vi "Measure IV AC.vi"(0 "IV Sampling":enum16{"Linear", "Logartihmic"}(ring)=enum."Logartihmic", 1 "6221 Address":string="12", 2 "SR860 Address":string="4", 5 "IV Type":T5(ring), 7 "dI or Imin":dbl=1e-08, 9 "Imax":dbl=0.001, 11 "Ipts":i16=16, 12 "Frequency":string="1711", 13 "Filter BW":T4(ring)=enum."10 ms", 14 "Ch1 Harmonic":T3(ring)) -> (8 "Data array":dbl[][](array[numeric])=[[1e-08, 3.5543477267321877e-09, 1.0096080012560406e-09, 0.35543477267321877, 0.10096080012560406], [2.1544e-08, 8.03021465434206e-08, 1.4967572525627115e-09, 3.727355483820117, 0.06947443615682841], [4.6416e-08, 1.2554884259996513e-07, 1.0072382615044234e-09, 2.704861310754161, 0.021700238312315226], [1e-07, 2.84475994760669e-07, 3.281983319934282e-09, 2.84475994760669, 0.03281983319934282], [2.15443e-07, 5.927384150172799e-07, 1.8001529832205674e-09, 2.7512539976572916, 0.00835558817515801], [4.64159e-07, 1.3026465262022668e-06, 1.3744287256216488e-09, 2.8064661596613805, 0.002961116181355201], [1e-06, 2.7703576330750934e-06, 1.1115718058886643e-09, 2.7703576330750934, 0.0011115718058886644], [2.154e-06, 5.988217456120992e-06, 6.723626581805896e-10, 2.780045244253014, 0.00031214608086378346], [4.642e-06, 1.3094926590184741e-05, 5.81885584849347e-10, 2.820966520935963, 0.00012535234486198772], [1e-05, 2.7790200547883614e-05, 2.9330275661149422e-09, 2.779020054788361, 0.0002933027566114942], [2.1544e-05, 5.994770525319382e-05, 3.4220733482770047e-10, 2.7825707971218816, 1.5884113202176964e-05], [4.6416e-05, 0.00012909908491565147, 1.8729144160359265e-09, 2.7813487787756697, 4.035062082118077e-05], [0.0001, 0.0002775546062139256, 2.9235413634973257e-09, 2.775546062139256, 2.9235413634973255e-05], [0.000215443, 0.0005982162022064585, 3.75564815539695e-09, 2.776679688857185, 1.7432212489600265e-05], [0.000464159, 0.001288317614580592, 1.080391628779838e-09, 2.7755954631507564, 2.3276326189513462e-06], [0.001, 0.00277545716289751, 3.798989931589336e-09, 2.77545716289751, 3.798989931589336e-06]], 10 "Error 6221":errorcluster, 15 "Error SR860":errorcluster)   [LabVIEW 2020]
uses:
  <vilib>/Analysis/1siggen.llb/Ramp Pattern by Delta.vi
  <vilib>/Analysis/NI_AALBase.lvlib
panel:
  out "I-V Plot":cluster{"Ramp Pattern":dbl[], dbl[]}[](graph)
  in  "TRIG Wave":bool=TRUE
  out "V STD Now":dbl=3.798989931589336e-09
  out "V Mean Now":dbl=0.00277545716289751
  out "Garbage":errorcluster={"status"=TRUE, "code"=6, "source"="GPIB Read in Measure IV.vi"}
  out "Lockin Garbage":string
  in  "Buffer Size (kb)":i32=2
  out "Buffer":sgl[](array[numeric])=[0.0027754628, 9.413887, 0.0027754628, 9.413885, 0.0027754628, 9.413885, 0.0027754628, 9.413884, 0.0027754628, 9.413881, 0.0027754628, 9.413881, 0.0027754628, 9.41388, 0.0027754628, 9.413878, 0.0027754628, 9.413878, 0.0027754626, 9.4138775, 0.0027754626, 9.4138775, 0.0027754626, 9.413875, 0.0027754626, 9.413875, 0.0027754626, 9.413874, 0.0027754626, 9.413872, 0.0027754626, 9.413872, 0.0027754626, 9.413871, 0.0027754626, 9.413868, 0.0027754626, 9.413868, 0.0027754626, 9.413866, 0.002775462, 9.413865, 0.002775462, 9.413865, 0.002775462, 9.413863, 0.002775462, 9.413863, 0.002775462, 9.413861, 0.002775462, 9.413859, 0.002775462, 9.413859, 0.0027754619, 9.413858, 0.0027754619, 9.413858, 0.0027754619, 9.4138565, 0.0027754619, 9.4138565, 0.0027754619, 9.413855, 0.0027754619, 9.413853, 0.0027754619, 9.413853, 0.0027754619, 9.41385, 0.0027754619, 9.41385, 0.0027754619, 9.41385, 0.0027754619, 9.413848, 0.0027754619, 9.413846, 0.0027754619, 9.413846, 0.0027754616, 9.413844, 0.0027754616, 9.413843, 0.0027754616, 9.413841, 0.0027754614, 9.413841, 0.0027754614, 9.413841, 0.0027754614, 9.413839, 0.0027754614, 9.413837, 0.0027754614, 9.413837, 0.0027754614, 9.4138365, 0.0027754614, 9.413835, 0.002775461, 9.413835, 0.002775461, 9.413835, 0.002775461, 9.413833, 0.002775461, 9.413831, 0.002775461, 9.413831, 0.002775461, 9.413828, 0.002775461, 9.413828, 0.002775461, 9.413828, 0.002775461, 9.413825, 0.002775461, 9.413824, 0.0027754607, 9.413824, 0.0027754607, 9.413822, 0.0027754607, 9.41382, 0.0027754607, 9.41382, 0.0027754605, 9.413818, 0.0027754605, 9.413818, 0.0027754605, 9.413817, 0.0027754605, 9.4138155, 0.0027754605, 9.4138155, 0.0027754605, 9.413814, 0.0027754605, 9.413812, 0.00277546, 9.413812, 0.00277546, 9.41381, 0.00277546, 9.413809, 0.00277546, 9.413809, 0.00277546, 9.413807, 0.0027754598, 9.413807, 0.0027754598, 9.413805, 0.0027754598, 9.413805, 0.0027754598, 9.413803, 0.0027754598, 9.413802, 0.0027754598, 9.413802, 0.0027754596, 9.413802, 0.0027754596, 9.413798, 0.0027754596, 9.413798, 0.0027754596, 9.413796, 0.0027754596, 9.413796, 0.0027754596, 9.413795, 0.0027754596, 9.413794, 0.0027754596, 9.413792, 0.0027754596, 9.413792, 0.0027754596, 9.41379, 0.0027754596, 9.413788, 0.0027754596, 9.413788, 0.0027754589, 9.413787, 0.0027754589, 9.413787, 0.0027754589, 9.413785, 0.0027754589, 9.413783, 0.0027754589, 9.413783, 0.0027754589, 9.413781, 0.0027754586, 9.413781, 0.0027754586, 9.41378, 0.0027754586, 9.413777, 0.0027754586, 9.413776, 0.0027754586, 9.4137745, 0.0027754586, 9.4137745, 0.0027754586, 9.413773, 0.0027754586, 9.413771, 0.0027754586, 9.413769, 0.0027754586, 9.413769, 0.0027754586, 9.413768, 0.0027754584, 9.413768, 0.0027754584, 9.413766, 0.0027754584, 9.413764, 0.0027754584, 9.413762, 0.0027754584, 9.413762, 0.0027754577, 9.413761, 0.0027754577, 9.413761, 0.0027754577, 9.413759, 0.0027754577, 9.413755, 0.0027754577, 9.413755, 0.0027754577, 9.4137535, 0.0027754577, 9.4137535, 0.0027754577, 9.413753, 0.0027754577, 9.413751, 0.0027754577, 9.413749, 0.0027754577, 9.413749, 0.0027754575, 9.413747, 0.0027754575, 9.413746, 0.0027754575, 9.413744, 0.0027754575, 9.413742, 0.0027754575, 9.41374, 0.0027754572, 9.41374, 0.0027754572, 9.413738, 0.0027754572, 9.413738, 0.0027754568, 9.413737, 0.0027754568, 9.413734, 0.0027754568, 9.4137335, 0.0027754568, 9.413732, 0.0027754568, 9.413731, 0.0027754568, 9.413731, 0.0027754568, 9.413728, 0.0027754568, 9.413727, 0.0027754565, 9.413727, 0.0027754565, 9.413725, 0.0027754565, 9.413724, 0.0027754565, 9.413721, 0.0027754565, 9.413719, 0.0027754563, 9.413718, 0.0027754563, 9.413718, 0.0027754563, 9.413716, 0.0027754563, 9.413714, 0.0027754563, 9.4137125, 0.002775456, 9.4137125, 0.002775456, 9.413712, 0.002775456, 9.413712, 0.002775456, 9.41371, 0.002775456, 9.413708, 0.0027754556, 9.413708, 0.0027754556, 9.413705, 0.0027754556, 9.413705, 0.0027754556, 9.413703, 0.0027754556, 9.413701, 0.0027754554, 9.413701, 0.0027754554, 9.413699, 0.0027754554, 9.413699, 0.0027754554, 9.413697, 0.0027754554, 9.413696, 0.0027754551, 9.413696, 0.0027754551, 9.413694, 0.0027754551, 9.413694, 0.0027754551, 9.413692, 0.0027754551, 9.413692, 0.0027754547, 9.413691, 0.0027754547, 9.41369, 0.0027754547, 9.413688, 0.0027754547, 9.413688, 0.0027754547, 9.413686, 0.0027754547, 9.413684, 0.0027754547, 9.413684, 0.0027754547, 9.413682, 0.0027754547, 9.413681, 0.0027754542, 9.413682, 0.0027754542, 9.413681, 0.0027754542, 9.413678, 0.0027754542, 9.413677, 0.0027754542, 9.413677, 0.002775454, 9.413677, 0.002775454, 9.413677, 0.002775454, 9.413673, 0.002775454, 9.413673, 0.002775454, 9.413673, 0.002775454, 9.4136715, 0.002775454, 9.4136715, 0.002775454, 9.413671, 0.002775454, 9.413671, 0.0027754535, 9.413671, 0.0027754535, 9.413669, 0.0027754535, 9.413667, 0.0027754535, 9.413667, 0.0027754535, 9.413665, 0.0027754533, 9.413667, 0.0027754533, 9.413665, 0.0027754533, 9.413663, 0.002775453, 9.413663, 0.002775453, 9.413663, 0.002775453, 9.413663, 0.002775453, 9.413662, 0.002775453, 9.413662, 0.002775453, 9.41366, 0.0027754526, 9.41366, 0.0027754526, 9.413658, 0.0027754526, 9.413658, 0.0027754526, 9.413658, 0.0027754523, 9.413658, 0.0027754523, 9.413656, 0.0027754523, 9.413656, 0.0027754523, 9.413656, 0.0027754523, 9.413655, 0.0027754523, 9.413655, 0.0027754523, 9.413655, 0.002775452, 9.413655, 0.002775452, 9.413653, 0.002775452, 9.413655, 0.002775452, 9.413653, 0.002775452, 9.413653, 0.002775452, 9.413653, 0.002775452, 9.413651, 0.0027754519, 9.413651, 0.0027754519, 9.413651, 0.0027754519, 9.413651, 0.0027754519, 9.41365, 0.0027754514, 9.413651, 0.0027754514, 9.413651, 0.0027754514, 9.41365, 0.0027754514, 9.41365, 0.0027754514, 9.41365, 0.0027754512, 9.41365, 0.0027754512, 9.41365, 0.0027754512, 9.41365, 0.0027754512, 9.413649, 0.0027754512, 9.41365, 0.0027754512, 9.41365, 0.0027754512, 9.413649, 0.0027754512, 9.413649, 0.002775451, 9.413649, 0.002775451, 9.413649, 0.002775451, 9.413649, 0.002775451, 9.413649, 0.0027754505, 9.413647, 0.0027754502, 9.413649, 0.0027754502, 9.413649, 0.0027754502, 9.413649, 0.0027754502, 9.413649, 0.0027754502, 9.413649, 0.0027754502, 9.413649]
  out "Buffer ASCII":string
  out "size(s)":i32=512
  out "R Buffer":sgl[](array[numeric])=[0.0027754628, 0.0027754628, 0.0027754628, 0.0027754628, 0.0027754628, 0.0027754628, 0.0027754628, 0.0027754628, 0.0027754628, 0.0027754626, 0.0027754626, 0.0027754626, 0.0027754626, 0.0027754626, 0.0027754626, 0.0027754626, 0.0027754626, 0.0027754626, 0.0027754626, 0.0027754626, 0.002775462, 0.002775462, 0.002775462, 0.002775462, 0.002775462, 0.002775462, 0.002775462, 0.0027754619, 0.0027754619, 0.0027754619, 0.0027754619, 0.0027754619, 0.0027754619, 0.0027754619, 0.0027754619, 0.0027754619, 0.0027754619, 0.0027754619, 0.0027754619, 0.0027754619, 0.0027754616, 0.0027754616, 0.0027754616, 0.0027754614, 0.0027754614, 0.0027754614, 0.0027754614, 0.0027754614, 0.0027754614, 0.0027754614, 0.002775461, 0.002775461, 0.002775461, 0.002775461, 0.002775461, 0.002775461, 0.002775461, 0.002775461, 0.002775461, 0.002775461, 0.0027754607, 0.0027754607, 0.0027754607, 0.0027754607, 0.0027754605, 0.0027754605, 0.0027754605, 0.0027754605, 0.0027754605, 0.0027754605, 0.0027754605, 0.00277546, 0.00277546, 0.00277546, 0.00277546, 0.00277546, 0.0027754598, 0.0027754598, 0.0027754598, 0.0027754598, 0.0027754598, 0.0027754598, 0.0027754596, 0.0027754596, 0.0027754596, 0.0027754596, 0.0027754596, 0.0027754596, 0.0027754596, 0.0027754596, 0.0027754596, 0.0027754596, 0.0027754596, 0.0027754596, 0.0027754589, 0.0027754589, 0.0027754589, 0.0027754589, 0.0027754589, 0.0027754589, 0.0027754586, 0.0027754586, 0.0027754586, 0.0027754586, 0.0027754586, 0.0027754586, 0.0027754586, 0.0027754586, 0.0027754586, 0.0027754586, 0.0027754586, 0.0027754584, 0.0027754584, 0.0027754584, 0.0027754584, 0.0027754584, 0.0027754577, 0.0027754577, 0.0027754577, 0.0027754577, 0.0027754577, 0.0027754577, 0.0027754577, 0.0027754577, 0.0027754577, 0.0027754577, 0.0027754577, 0.0027754575, 0.0027754575, 0.0027754575, 0.0027754575, 0.0027754575, 0.0027754572, 0.0027754572, 0.0027754572, 0.0027754568, 0.0027754568, 0.0027754568, 0.0027754568, 0.0027754568, 0.0027754568, 0.0027754568, 0.0027754568, 0.0027754565, 0.0027754565, 0.0027754565, 0.0027754565, 0.0027754565, 0.0027754563, 0.0027754563, 0.0027754563, 0.0027754563, 0.0027754563, 0.002775456, 0.002775456, 0.002775456, 0.002775456, 0.002775456, 0.0027754556, 0.0027754556, 0.0027754556, 0.0027754556, 0.0027754556, 0.0027754554, 0.0027754554, 0.0027754554, 0.0027754554, 0.0027754554, 0.0027754551, 0.0027754551, 0.0027754551, 0.0027754551, 0.0027754551, 0.0027754547, 0.0027754547, 0.0027754547, 0.0027754547, 0.0027754547, 0.0027754547, 0.0027754547, 0.0027754547, 0.0027754547, 0.0027754542, 0.0027754542, 0.0027754542, 0.0027754542, 0.0027754542, 0.002775454, 0.002775454, 0.002775454, 0.002775454, 0.002775454, 0.002775454, 0.002775454, 0.002775454, 0.002775454, 0.0027754535, 0.0027754535, 0.0027754535, 0.0027754535, 0.0027754535, 0.0027754533, 0.0027754533, 0.0027754533, 0.002775453, 0.002775453, 0.002775453, 0.002775453, 0.002775453, 0.002775453, 0.0027754526, 0.0027754526, 0.0027754526, 0.0027754526, 0.0027754523, 0.0027754523, 0.0027754523, 0.0027754523, 0.0027754523, 0.0027754523, 0.0027754523, 0.002775452, 0.002775452, 0.002775452, 0.002775452, 0.002775452, 0.002775452, 0.002775452, 0.0027754519, 0.0027754519, 0.0027754519, 0.0027754519, 0.0027754514, 0.0027754514, 0.0027754514, 0.0027754514, 0.0027754514, 0.0027754512, 0.0027754512, 0.0027754512, 0.0027754512, 0.0027754512, 0.0027754512, 0.0027754512, 0.0027754512, 0.002775451, 0.002775451, 0.002775451, 0.002775451, 0.0027754505, 0.0027754502, 0.0027754502, 0.0027754502, 0.0027754502, 0.0027754502, 0.0027754502]
  out "Theta Buffer":sgl[](array[numeric])=[9.413887, 9.413885, 9.413885, 9.413884, 9.413881, 9.413881, 9.41388, 9.413878, 9.413878, 9.4138775, 9.4138775, 9.413875, 9.413875, 9.413874, 9.413872, 9.413872, 9.413871, 9.413868, 9.413868, 9.413866, 9.413865, 9.413865, 9.413863, 9.413863, 9.413861, 9.413859, 9.413859, 9.413858, 9.413858, 9.4138565, 9.4138565, 9.413855, 9.413853, 9.413853, 9.41385, 9.41385, 9.41385, 9.413848, 9.413846, 9.413846, 9.413844, 9.413843, 9.413841, 9.413841, 9.413841, 9.413839, 9.413837, 9.413837, 9.4138365, 9.413835, 9.413835, 9.413835, 9.413833, 9.413831, 9.413831, 9.413828, 9.413828, 9.413828, 9.413825, 9.413824, 9.413824, 9.413822, 9.41382, 9.41382, 9.413818, 9.413818, 9.413817, 9.4138155, 9.4138155, 9.413814, 9.413812, 9.413812, 9.41381, 9.413809, 9.413809, 9.413807, 9.413807, 9.413805, 9.413805, 9.413803, 9.413802, 9.413802, 9.413802, 9.413798, 9.413798, 9.413796, 9.413796, 9.413795, 9.413794, 9.413792, 9.413792, 9.41379, 9.413788, 9.413788, 9.413787, 9.413787, 9.413785, 9.413783, 9.413783, 9.413781, 9.413781, 9.41378, 9.413777, 9.413776, 9.4137745, 9.4137745, 9.413773, 9.413771, 9.413769, 9.413769, 9.413768, 9.413768, 9.413766, 9.413764, 9.413762, 9.413762, 9.413761, 9.413761, 9.413759, 9.413755, 9.413755, 9.4137535, 9.4137535, 9.413753, 9.413751, 9.413749, 9.413749, 9.413747, 9.413746, 9.413744, 9.413742, 9.41374, 9.41374, 9.413738, 9.413738, 9.413737, 9.413734, 9.4137335, 9.413732, 9.413731, 9.413731, 9.413728, 9.413727, 9.413727, 9.413725, 9.413724, 9.413721, 9.413719, 9.413718, 9.413718, 9.413716, 9.413714, 9.4137125, 9.4137125, 9.413712, 9.413712, 9.41371, 9.413708, 9.413708, 9.413705, 9.413705, 9.413703, 9.413701, 9.413701, 9.413699, 9.413699, 9.413697, 9.413696, 9.413696, 9.413694, 9.413694, 9.413692, 9.413692, 9.413691, 9.41369, 9.413688, 9.413688, 9.413686, 9.413684, 9.413684, 9.413682, 9.413681, 9.413682, 9.413681, 9.413678, 9.413677, 9.413677, 9.413677, 9.413677, 9.413673, 9.413673, 9.413673, 9.4136715, 9.4136715, 9.413671, 9.413671, 9.413671, 9.413669, 9.413667, 9.413667, 9.413665, 9.413667, 9.413665, 9.413663, 9.413663, 9.413663, 9.413663, 9.413662, 9.413662, 9.41366, 9.41366, 9.413658, 9.413658, 9.413658, 9.413658, 9.413656, 9.413656, 9.413656, 9.413655, 9.413655, 9.413655, 9.413655, 9.413653, 9.413655, 9.413653, 9.413653, 9.413653, 9.413651, 9.413651, 9.413651, 9.413651, 9.41365, 9.413651, 9.413651, 9.41365, 9.41365, 9.41365, 9.41365, 9.41365, 9.41365, 9.413649, 9.41365, 9.41365, 9.413649, 9.413649, 9.413649, 9.413649, 9.413649, 9.413649, 9.413647, 9.413649, 9.413649, 9.413649, 9.413649, 9.413649, 9.413649]
  out "#n":string="#4"
  out "cccc":string="2048"
  out "number of bytes":i32=2048
  out "n":i32=4
  out "CaptureStat":i32=6
  out "Current Now":string="1.000E-3"
  in  "stop":bool
  in  "Measure?":bool=TRUE
  out "IRNG":string="2\n"
  out "IRNG Now":dbl=0.1
  out "SCAL Now":dbl=0.02
  out "SCAL":string="20\n"
  out "OFLT LUT":dbl[](array[numeric])=[1e-06, 3e-06, 1e-05, 3e-05, 0.0001, 0.0003, 0.001, 0.003, 0.01, 0.03, 0.1, 0.3, 1.0, 3.0, 10.0, 30.0, 100.0, 300.0, 1000.0, 3000.0, 10000.0, 30000.0]
  out "SCAL LUT":dbl[](array[numeric])=[1.0, 0.5, 0.2, 0.1, 0.05, 0.02, 0.01, 0.005, 0.002, 0.001, 0.0005, 0.0002, 0.0001, 5e-05, 2e-05, 1e-05, 5e-06, 2e-06, 1e-06, 5e-07, 2e-07, 1e-07, 5e-08, 2e-08, 1e-08, 5e-09, 2e-09, 1e-09]
  out "IRNG LUT":dbl[](array[numeric])=[1.0, 0.3, 0.1, 0.03, 0.01]
  out "Input Range":T1(ring)=enum."100 mV"
  out "Sensitivity":T2(ring)=enum."20 mV"
  in  "Buffer Data":enum16{"X", "XY", "RT", "XYRT"}(ring)=enum."RT"
  in  "Rate decimation":i32=1
  out "SR860 Commands":string="*RST;\nIVMD VOLTAGE;\nISRC A-B;\nICPL AC;\nIGND GROund;\nSYNC OFF;\nOFSL 3;\nOFLT 8;\nRSRC EXT;\nRTRG NEGttl;\nREFZ 1Meg;\nHARM 1;\nARNG;\nASCL;\nAPHS;\nASCL;\nCAPTURELEN 2;\nCAPTURECFG 2;\nCAPTURERATE 1;\n"
  out "6221 Range":dbl=0.001
  in  "INIT 6221":bool=TRUE
  out "6221 Commands":string="*RST\nTRIG:OLIN 4\nOUTP:LTEarth ON\nCURR:RANG 100.000E-9\nSOUR:WAVE:AMPL 10.000E-9\nSOUR:WAVE:FREQ 1711\nSOUR:WAVE:FUNC SIN\nSOUR:WAVE:OFFS 0\nSOUR:WAVE:PMAR:STAT ON\nSOUR:WAVE:PMAR:OLIN 2\nSOUR:WAVE:RANG FIXED\nSOUR:CURR:COMP 25\nSOUR:WAVE:ARM\nSOUR:WAVE:INIT"
  out "Current Samples":dbl[](array[numeric])=[1e-08, 2.154434690031884e-08, 4.641588833612779e-08, 1e-07, 2.1544346900318832e-07, 4.6415888336127773e-07, 1e-06, 2.1544346900318822e-06, 4.641588833612778e-06, 1e-05, 2.1544346900318823e-05, 4.641588833612778e-05, 0.0001, 0.00021544346900318823, 0.00046415888336127724, 0.001]
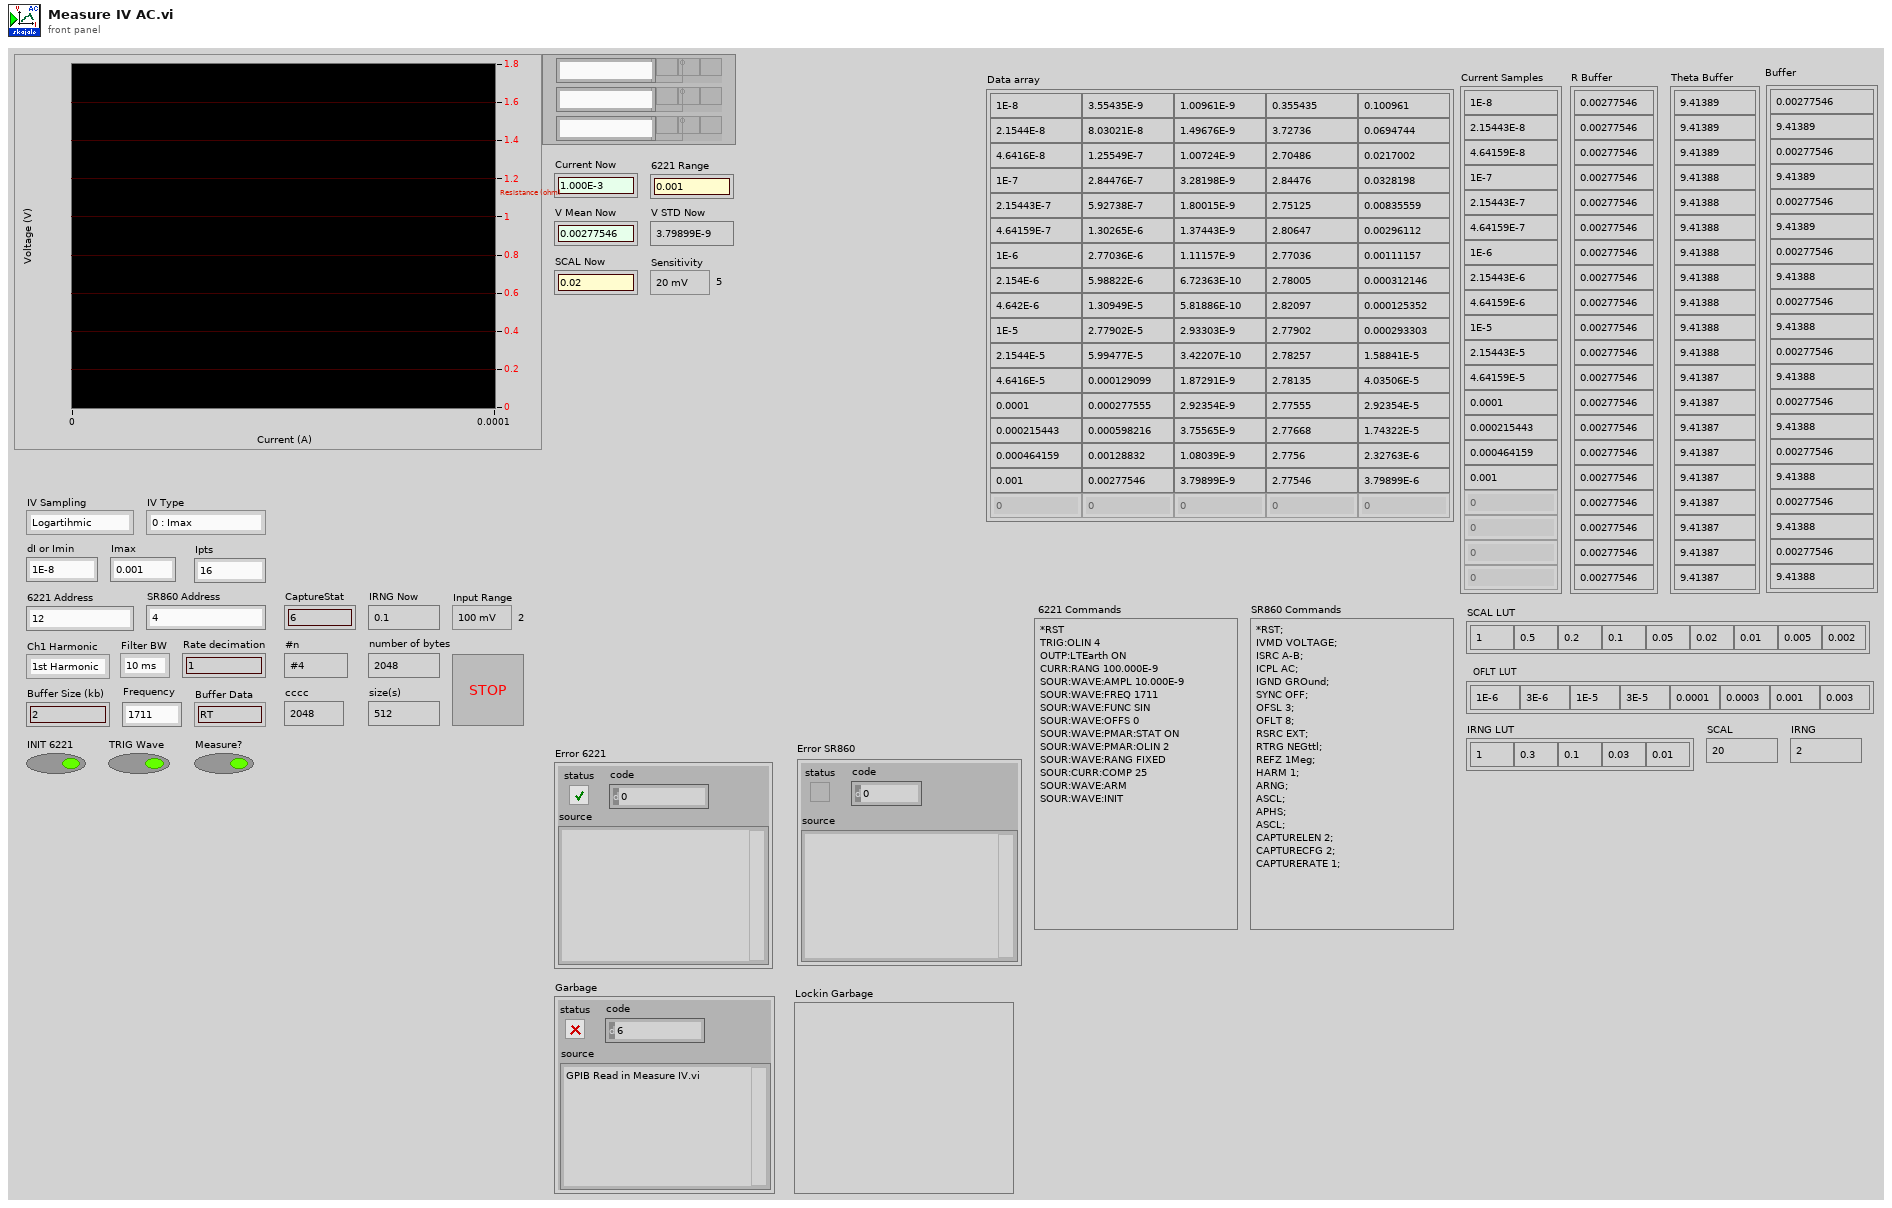
[diagram p1: front panel]
types:
  T1 = enum16{"1 V", "300 mV", "100 mV", "30 mV", "10 mV"}
  T2 = enum16{"1 V", "500 mV", "200 mV", "100 mV", "50 mV", "20 mV", "10 mV", "5 mV", "2 mV", "1 mV", "500 uV", "200 uV", "100 uV", "50 uV", "20 uV", "10 uV", "5 uV", "2 uV", "1 uV", "500 nV", "200 nV", "100 nV", "50 nV", "20 nV", "10 nV", "5 nV", "2 nV", "1 nV"}
  T3 = enum16{"1st Harmonic", "2nd Harmonic", "3rd Harmonic"}
  T4 = enum16{"1 us", "3 us", "10 us", "30 us", "100 us", "300 us", "1 ms", "3 ms", "10 ms", "30 ms", "100 ms", "300 ms", "1 s", "3 s", "10 s", "30 s", "100 s", "300 s"}
  T5 = enum16{"0 : Imax", "0 : Imax : 0", "0 : Imax : -Imax : 0"}
  T6 = enum16{"big-endian, network order", "native, host order", "little-endian"}
  T7 = cluster{"Data array":dbl[], "Data array":dbl[]}[]
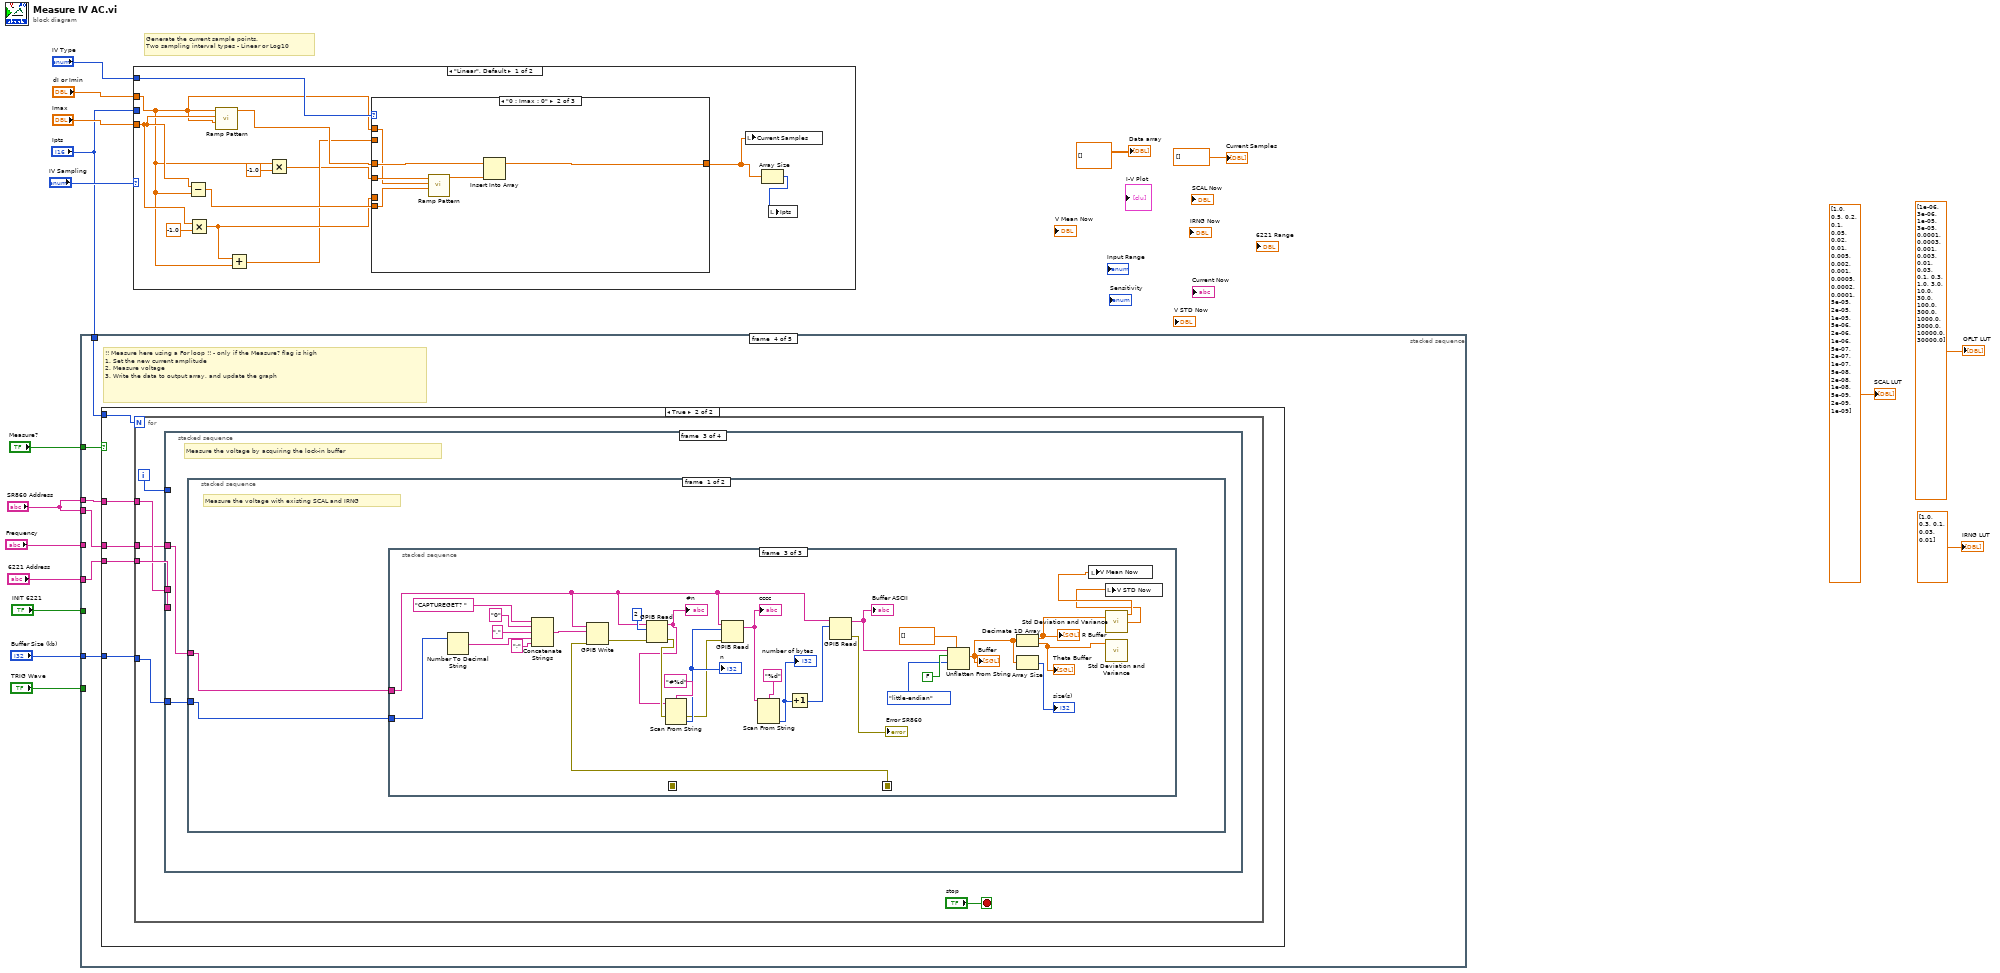
[diagram p0: block diagram]
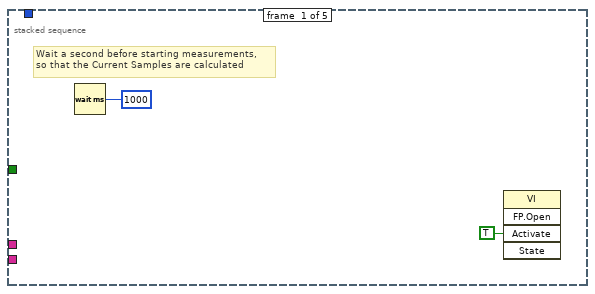
[diagram p2: hidden frame]
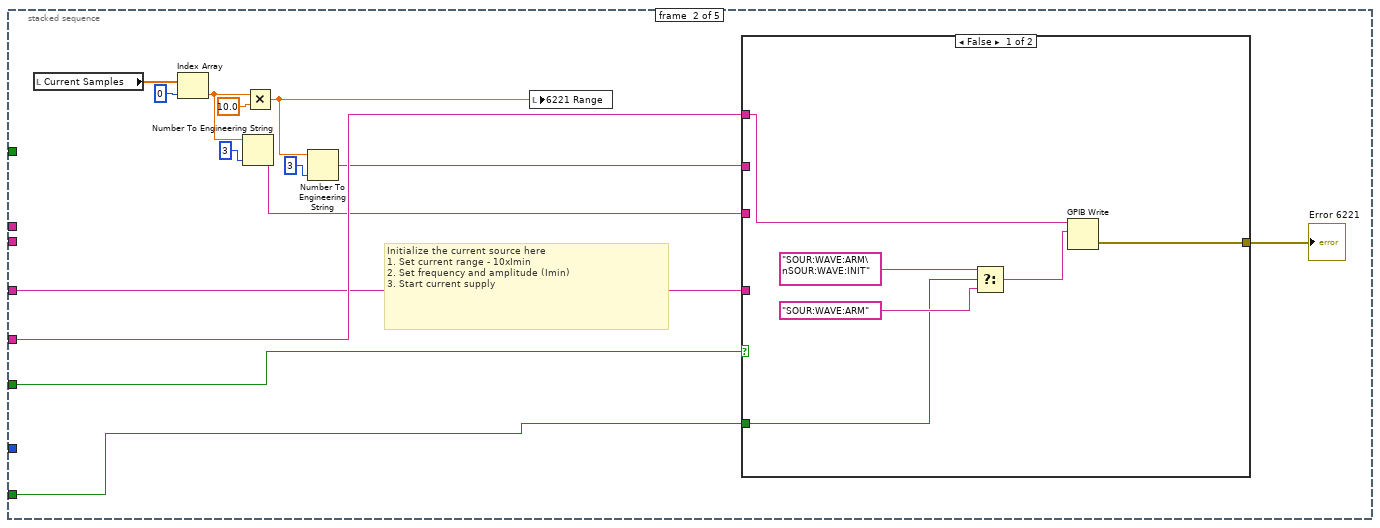
[diagram p3: hidden frame]
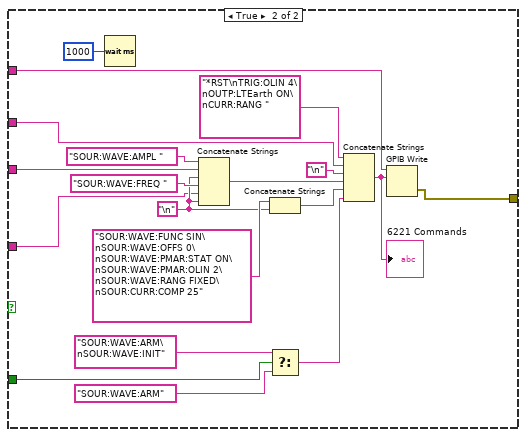
[diagram p4: hidden frame]
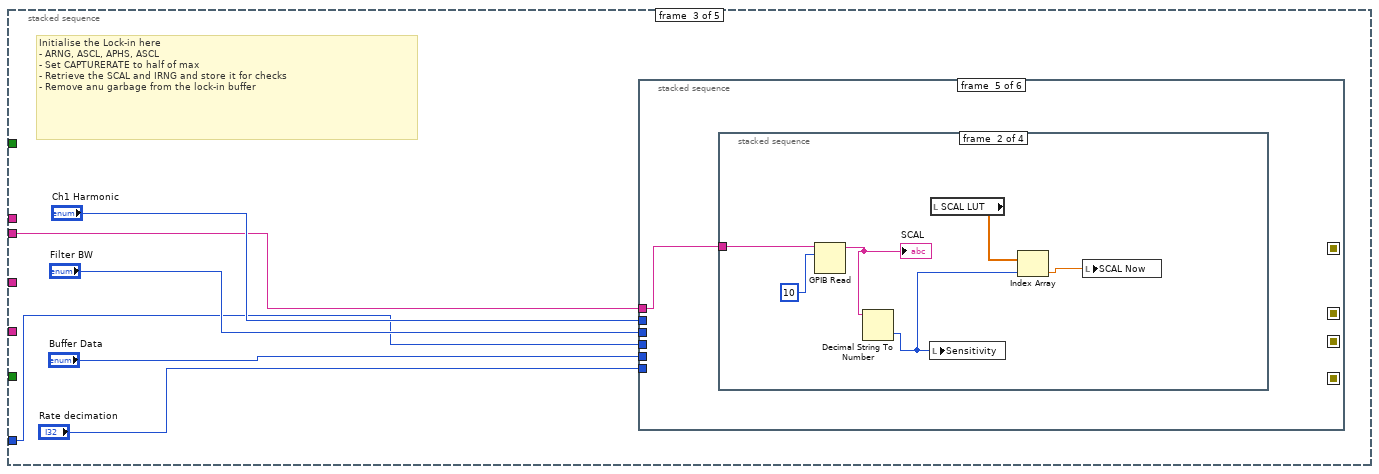
[diagram p5: hidden frame]
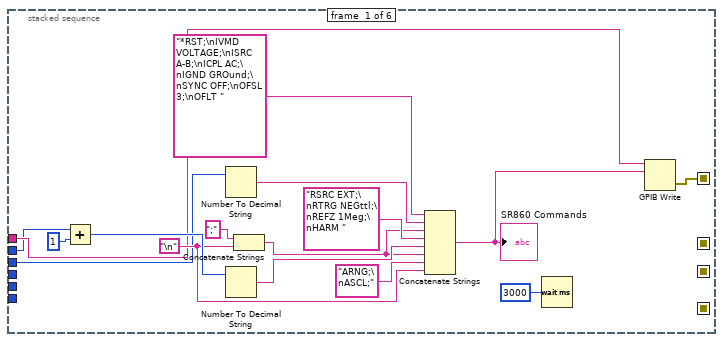
[diagram p6: hidden frame]
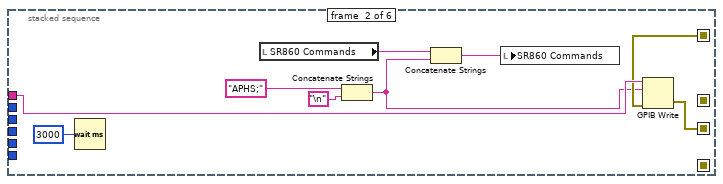
[diagram p7: hidden frame]
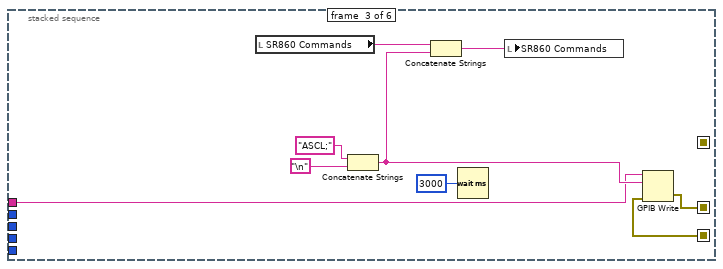
[diagram p8: hidden frame]
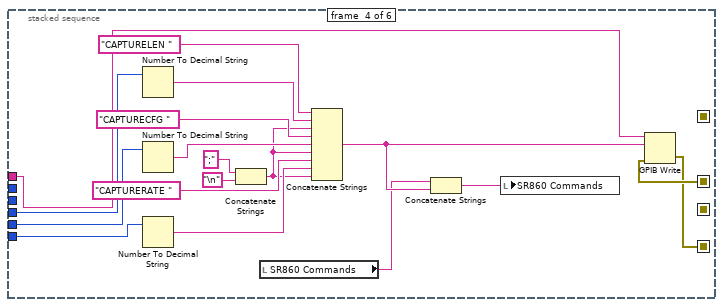
[diagram p9: hidden frame]
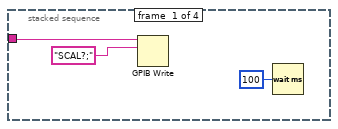
[diagram p10: hidden frame]
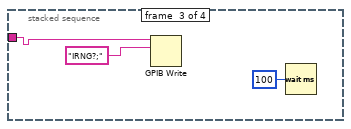
[diagram p11: hidden frame]
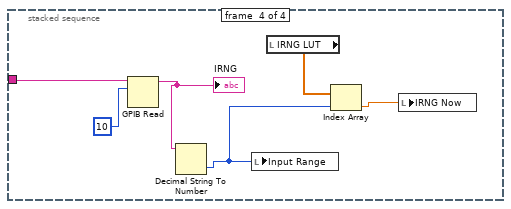
[diagram p12: hidden frame]
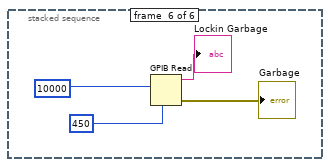
[diagram p13: hidden frame]
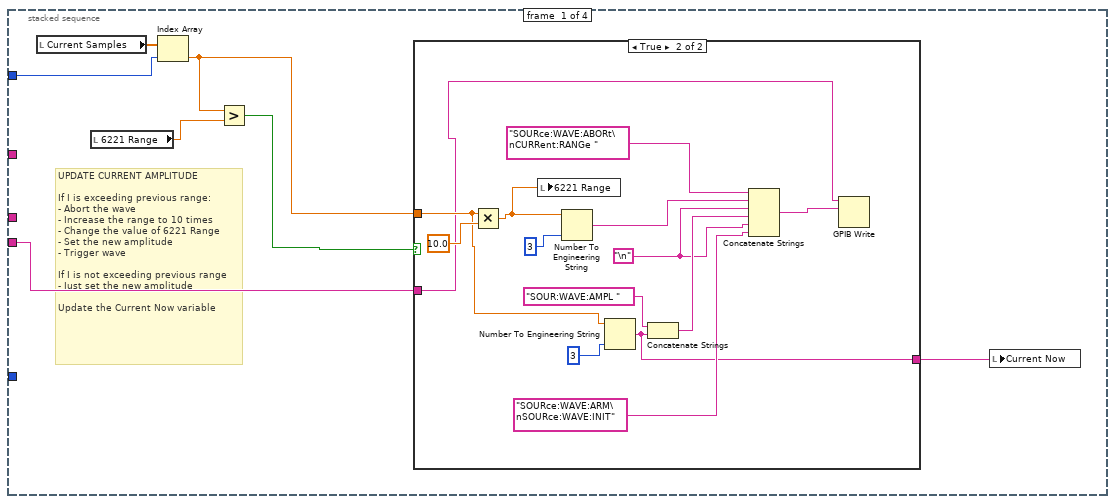
[diagram p15: hidden frame]
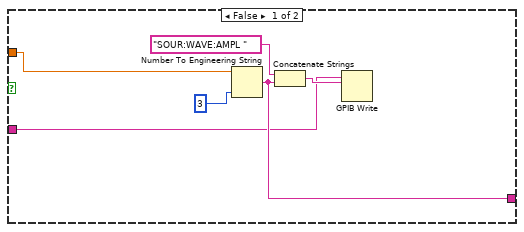
[diagram p16: hidden frame]
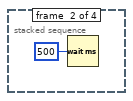
[diagram p17: hidden frame]
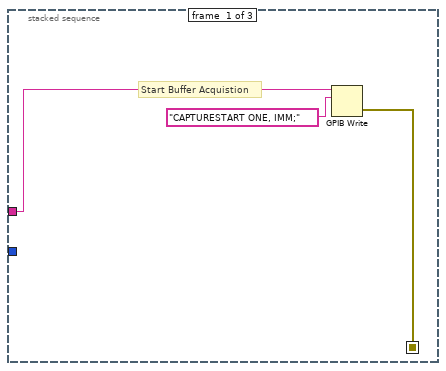
[diagram p18: hidden frame]
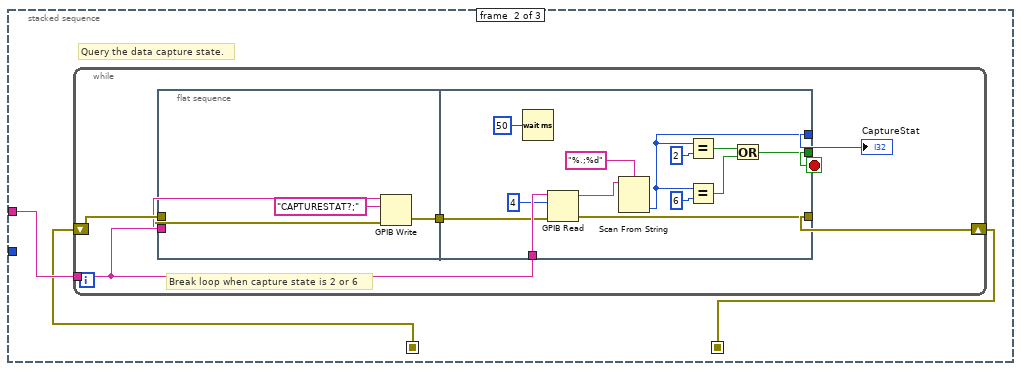
[diagram p19: hidden frame]
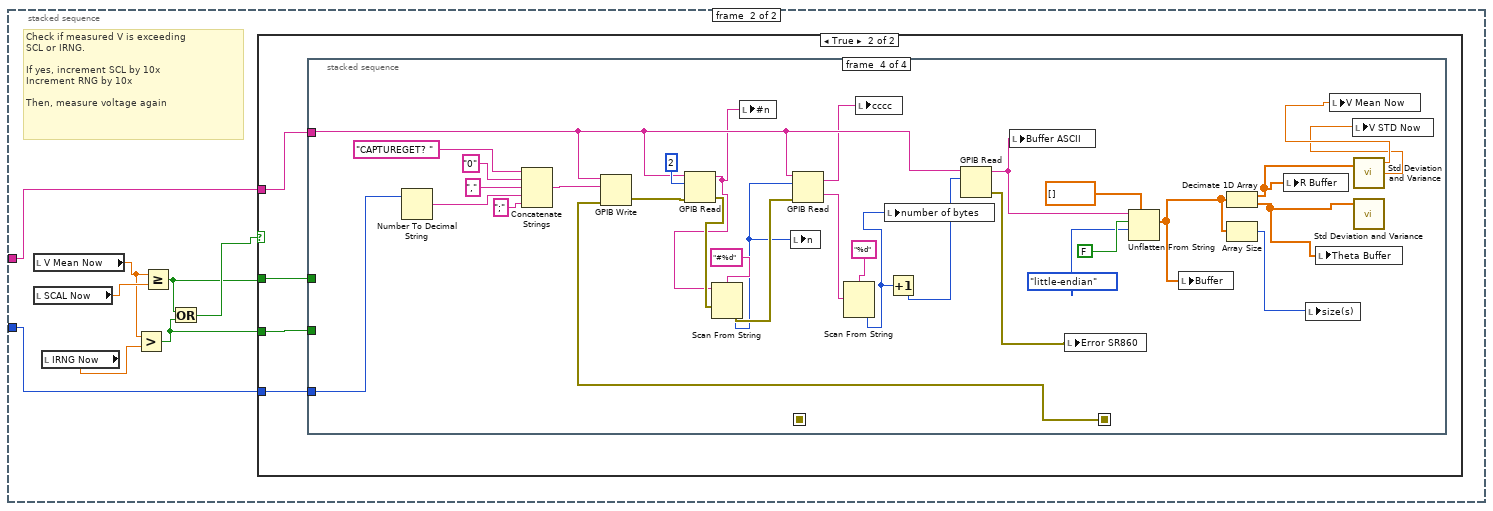
[diagram p20: hidden frame]
diagram:
  # "Generate the current sample points.\nTwo sampling interval types - Linear or Log10"
  n1 = stacked-sequence {
    tunnel: "INIT 6221" -> [_ w33 _ _ _]
    tunnel: "6221 Address" -> [_ w32 _ w143 w378]
    tunnel: "Frequency" -> [_ w31 _ _ _]
    tunnel: "SR860 Address" -> [_ _ w60 w142 _]
    tunnel: "Measure?" -> [_ _ _ w145 _]
    tunnel: "Ipts" -> [_ _ _ w144 _]
    tunnel: "SR860 Address" -> [_ _ _ w141 _]
    tunnel: "Buffer Size (kb)" -> [_ _ w59 w140 _]
    tunnel: "TRIG Wave" -> [_ w20 _ _ _]
    frame #0 {
      # "Wait a second before starting measurements,\nso that the Current Samples are calculated"
      n2 = Wait (ms)(milliseconds to wait=u32 1000) -> ()  [unwired: 1 out]
      n3 = invoke class="VI" method="FP.Open"("Activate"=TRUE ("Activate?")) -> ()  [unwired: 4 in, 5 out]
    }
    frame #1 {
      # "Initialize the current source here\n1. Set current range - 10xImin\n2. Set frequency and amplitude (Imin)\n3. Start current supply"
      n4 = local read "Current Samples"() -> (w30:dbl[])
      n5 = Index Array(array=w30, index=0) -> (element=w27:dbl)
      n6 = Number To Engineering String(2:i16 3 ("precision (6)"), 4:w27) -> (0:w28:string)  [unwired: 2 in]
      n7 = Multiply(x=w27, y=10.0) -> (x*y=w22:dbl)
      n8 = Number To Engineering String(2:i16 3 ("precision (6)"), 4:w22) -> (0:w25:string)  [unwired: 2 in]
      n9 = local write "6221 Range"(w22) -> ()
      n10 = case shown="False" w33 {
        tunnel: w32 -> [w38 w46]
        tunnel: w31 -> [_ w45]
        tunnel: w28 -> [_ w44]
        tunnel: w25 -> [_ w42]
        tunnel: [w39 w41] -> w21
        tunnel: w20 -> [w35 w40]
        frame False {
          n11 = Select(t="SOUR:WAVE:ARM\nSOUR:WAVE:INIT" ("string"), s=w35, f="SOUR:WAVE:ARM" ("string")) -> (s? t:f=w34:string)
          n12 = GPIB Write(0:w38, 1:w34) -> (6:w39:errorcluster)  [unwired: 3 in, 1 out]
        }
        frame True {
          w48 = "\n"
          n13 = Wait (ms)(milliseconds to wait=u32 1000) -> ()  [unwired: 1 out]
          n14 = Concatenate Strings("SOUR:WAVE:AMPL ", w44, w48, "SOUR:WAVE:FREQ ", w45, w48) -> (w55:string)
          n15 = Concatenate Strings("SOUR:WAVE:FUNC SIN\nSOUR:WAVE:OFFS 0\nSOUR:WAVE:PMAR:STAT ON\nSOUR:WAVE:PMAR:OLIN 2\nSOUR:WAVE:RANG FIXED\nSOUR:CURR:COMP 25", w48) -> (w54:string)
          n16 = Select(t="SOUR:WAVE:ARM\nSOUR:WAVE:INIT" ("string"), s=w40, f="SOUR:WAVE:ARM" ("string")) -> (s? t:f=w51:string)
          n17 = Concatenate Strings("*RST\nTRIG:OLIN 4\nOUTP:LTEarth ON\nCURR:RANG ", w42, "\n", w55, w54, w51) -> (w53:string)
          "6221 Commands" <- w53
          n18 = GPIB Write(0:w46, 1:w53) -> (6:w41:errorcluster)  [unwired: 3 in, 1 out]
        }
      }
      "Error 6221" <- w21
    }
    frame #2 {
      # "Initialise the Lock-in here\n- ARNG, ASCL, APHS, ASCL\n- Set CAPTURERATE to half of max\n- Retrieve the SCAL and IRNG and store it for checks\n- Remove anu garbage from the lock-in buffer"
      n19 = stacked-sequence {
        seq-local: [w67 _ _ _ _ _] -> [_ w88 _ _ _ _]
        seq-local: [_ w87 _ _ _ _] -> [_ _ w92 _ _ _]
        seq-local: [_ _ w90 _ _ _] -> [_ _ _ w100 _ _]
        seq-local: [_ _ _ w99 _ _] -> [_ _ _ _ _ _]
        tunnel: w60 -> [w68 w89 w93 w107 w117 _]
        tunnel: "Rate decimation" -> [_ _ _ w103 _ _]
        tunnel: "Buffer Data" -> [_ _ _ w102 _ _]
        tunnel: w59 -> [_ _ _ w101 _ _]
        tunnel: "Filter BW" -> [w66 _ _ _ _ _]
        tunnel: "Ch1 Harmonic" -> [w65 _ _ _ _ _]
        frame #0 {
          w71 = "\n"
          n20 = Add(x=w65, y=1) -> (x+y=w74:i32)
          n21 = Number To Decimal String(number=w66) -> (decimal integer string=w79:string)  [unwired: 1 in]
          n22 = Number To Decimal String(number=w74) -> (decimal integer string=w76:string)  [unwired: 1 in]
          n23 = Concatenate Strings(";" ("string"), w71) -> (w75:string)
          n24 = Concatenate Strings("*RST;\nIVMD VOLTAGE;\nISRC A-B;\nICPL AC;\nIGND GROund;\nSYNC OFF;\nOFSL 3;\nOFLT ", w79, w75, "RSRC EXT;\nRTRG NEGttl;\nREFZ 1Meg;\nHARM ", w76, w75, "ARNG;\nASCL;", w71) -> (w69:string)
          "SR860 Commands" <- w69
          n25 = Wait (ms)(milliseconds to wait=u32 3000) -> ()  [unwired: 1 out]
          n26 = GPIB Write(0:w68, 1:w69) -> (6:w67:errorcluster)  [unwired: 3 in, 1 out]
        }
        frame #1 {
          n27 = Wait (ms)(milliseconds to wait=u32 3000) -> ()  [unwired: 1 out]
          n28 = local read "SR860 Commands"() -> (w83:string)
          n29 = Concatenate Strings("APHS;", "\n") -> (w84:string)
          n30 = Concatenate Strings(w83, w84) -> (w82:string)
          n31 = local write "SR860 Commands"(w82) -> ()
          n32 = GPIB Write(0:w89, 1:w84, 3:w88) -> (6:w87:errorcluster)  [unwired: 2 in, 1 out]
        }
        frame #2 {
          n33 = local read "SR860 Commands"() -> (w95:string)
          n34 = Concatenate Strings("ASCL;", "\n") -> (w96:string)
          n35 = Concatenate Strings(w95, w96) -> (w94:string)
          n36 = Wait (ms)(milliseconds to wait=u32 3000) -> ()  [unwired: 1 out]
          n37 = local write "SR860 Commands"(w94) -> ()
          n38 = GPIB Write(0:w93, 1:w96, 3:w92) -> (6:w90:errorcluster)  [unwired: 2 in, 1 out]
        }
        frame #3 {
          n39 = Number To Decimal String(number=w101) -> (decimal integer string=w115:string)  [unwired: 1 in]
          n40 = Number To Decimal String(number=w102) -> (decimal integer string=w112:string)  [unwired: 1 in]
          n41 = Number To Decimal String(number=w103) -> (decimal integer string=w109:string)  [unwired: 1 in]
          n42 = Concatenate Strings(";" ("string"), "\n") -> (w108:string)
          n43 = local read "SR860 Commands"() -> (w104:string)
          n44 = Concatenate Strings("CAPTURELEN ", w115, w108, "CAPTURECFG ", w112, w108, "CAPTURERATE ", w109, w108) -> (w106:string)
          n45 = Concatenate Strings(w104, w106) -> (w105:string)
          n46 = local write "SR860 Commands"(w105) -> ()
          n47 = GPIB Write(0:w107, 1:w106, 3:w100) -> (6:w99:errorcluster)  [unwired: 2 in, 1 out]
        }
        frame #4 {
          n48 = stacked-sequence {
            tunnel: w117 -> [w119 w124 w127 w133]
            frame #0 {
              n49 = GPIB Write(0:w119, 1:"SCAL?;" ("data")) -> ()  [unwired: 3 in, 2 out]
              n50 = Wait (ms)(milliseconds to wait=u32 100) -> ()  [unwired: 1 out]
            }
            frame #1 {
              n51 = GPIB Read(0:w124, 1:10 ("byte count")) -> (5:w125:string)  [unwired: 3 in, 2 out]
              "SCAL" <- w125
              n52 = Decimal String To Number(string=w125) -> (number=w122:i32)  [unwired: 2 in, 1 out]
              n53 = local write "Sensitivity"(w122) -> ()
              n54 = local read "SCAL LUT"() -> (w123:dbl[])
              n55 = Index Array(array=w123, index=w122) -> (element=w121:dbl)
              n56 = local write "SCAL Now"(w121) -> ()
            }
            frame #2 {
              n57 = GPIB Write(0:w127, 1:"IRNG?;" ("data")) -> ()  [unwired: 3 in, 2 out]
              n58 = Wait (ms)(milliseconds to wait=u32 100) -> ()  [unwired: 1 out]
            }
            frame #3 {
              n59 = GPIB Read(0:w133, 1:10 ("byte count")) -> (5:w134:string)  [unwired: 3 in, 2 out]
              "IRNG" <- w134
              n60 = Decimal String To Number(string=w134) -> (number=w130:i32)  [unwired: 2 in, 1 out]
              n61 = local write "Input Range"(w130) -> ()
              n62 = local read "IRNG LUT"() -> (w131:dbl[])
              n63 = Index Array(array=w131, index=w130) -> (element=w132:dbl)
              n64 = local write "IRNG Now"(w132) -> ()
            }
          }
        }
        frame #5 {
          n65 = GPIB Read(1:10000 ("byte count"), 4:450 ("timeout ms (488.2 global)")) -> (5:→"Lockin Garbage":string, 7:→"Garbage":errorcluster)  [unwired: 3 in, 1 out]
        }
      }
    }
    frame #3 {
      # "!! Measure here using a For loop !! - only if the Measure? flag is high\n1. Set the new current amplitude\n2. Measure voltage\n3. Write the data to output array, and update the graph"
      n66 = case shown="True" w145 {
        tunnel: w144 -> [_ w150]
        tunnel: w143 -> [_ w149]
        tunnel: w142 -> [_ w148]
        tunnel: w141 -> [_ w147]
        tunnel: w140 -> [_ w146]
        frame False {
        }
        frame True {
          n67 = for {
            N: w150 -> [_]
            tunnel: w149 -> [w154]
            tunnel: w148 -> [w153]
            tunnel: w147 -> [w152]
            tunnel: w146 -> [w151]
            i -> [w155]
            stop <- "stop" stop-if-true
            n68 = stacked-sequence {
              tunnel: w155 -> [w162 _ _ _]
              tunnel: w154 -> [w157 _ _ _]
              tunnel: w153 -> [_ _ _ _]
              tunnel: w152 -> [_ _ w186 _]
              tunnel: w151 -> [_ _ w185 _]
              frame #0 {
                # "UPDATE CURRENT AMPLITUDE\n\nIf I is exceeding previous range:\n- Abort the wave\n- Increase the range to 10 times\n- Change the value of 6221 Range\n- Set the new amplitude\n- Trigger wave\n\nIf I is not exceeding previous range\n- Just set the new amplitude\n\nUpdate the Current Now variable"
                n69 = local read "Current Samples"() -> (w163:dbl[])
                n70 = local read "6221 Range"() -> (w161:dbl)
                n71 = Index Array(array=w163, index=w162) -> (element=w159:dbl)
                n72 = Greater?(x=w159, y=w161) -> (0:w160:bool)
                n73 = case shown="True" w160 {
                  tunnel: w159 -> [w166 w176]
                  tunnel: [w165 w171] -> w158
                  tunnel: w157 -> [w164 w170]
                  frame False {
                    n74 = Number To Engineering String(2:i16 3 ("precision (6)"), 4:w166) -> (0:w165:string)  [unwired: 2 in]
                    n75 = Concatenate Strings("SOUR:WAVE:AMPL " ("string"), w165) -> (w167:string)
                    n76 = GPIB Write(0:w164, 1:w167) -> ()  [unwired: 3 in, 2 out]
                  }
                  frame True {
                    w174 = "\n"
                    n77 = Multiply(x=w176, y=10.0) -> (x*y=w172:dbl)
                    n78 = local write "6221 Range"(w172) -> ()
                    n79 = Number To Engineering String(2:i16 3 ("precision (6)"), 4:w172) -> (0:w179:string)  [unwired: 2 in]
                    n80 = Number To Engineering String(2:i16 3 ("precision (6)"), 4:w176) -> (0:w171:string)  [unwired: 2 in]
                    n81 = Concatenate Strings("SOUR:WAVE:AMPL " ("string"), w171) -> (w175:string)
                    n82 = Concatenate Strings("SOURce:WAVE:ABORt\nCURRent:RANGe " ("string"), w179, w174, w175, w174, "SOURce:WAVE:ARM\nSOURce:WAVE:INIT" ("string")) -> (w183:string)
                    n83 = GPIB Write(0:w170, 1:w183) -> ()  [unwired: 3 in, 2 out]
                  }
                }
                n84 = local write "Current Now"(w158) -> ()
              }
              frame #1 {
                n85 = Wait (ms)(milliseconds to wait=u32 500) -> ()  [unwired: 1 out]
              }
              frame #2 {
                # "Measure the voltage by acquiring the lock-in buffer"
                n86 = stacked-sequence {
                  tunnel: w186 -> [w188 w256]
                  tunnel: w185 -> [w187 w255]
                  frame #0 {
                    # "Measure the voltage with existing SCAL and IRNG"
                    n87 = stacked-sequence {
                      seq-local: [_ w193 _] -> [_ _ w220]
                      seq-local: [w189 _ _] -> [_ w192 _]
                      tunnel: w188 -> [w191 w194 w222]
                      tunnel: w187 -> [_ _ w226]
                      frame #0 {
                        # "Start Buffer Acquistion"
                        n88 = GPIB Write(0:w191, 1:"CAPTURESTART ONE, IMM;" ("data")) -> (6:w189:errorcluster)  [unwired: 3 in, 1 out]
                      }
                      frame #1 {
                        # "Query the data capture state."
                        n89 = while {
                          tunnel: w194 -> [w199]
                          shift-right: [w195] -> w193
                          shift-left: w192 -> [w196]
                          stop <- w198 stop-if-true
                          # "Break loop when capture state is 2 or 6"
                          n90 = flat-sequence {
                            tunnel: w199 -> [w202]
                            tunnel: [w203] -> w200
                            tunnel: w196 -> [w201]
                            tunnel: w200 -> [w210]
                            tunnel: w199 -> [w212]
                            tunnel: [w208] -> w198
                            tunnel: [w207] -> w197
                            tunnel: [w205] -> w195
                            frame #0 {
                              n91 = GPIB Write(0:w202, 1:"CAPTURESTAT?;", 3:w201) -> (6:w203:errorcluster)  [unwired: 2 in, 1 out]
                            }
                            frame #1 {
                              n92 = Wait (ms)(milliseconds to wait=u32 50) -> ()  [unwired: 1 out]
                              n93 = GPIB Read(0:w212, 1:u32 4 ("byte count"), 3:w210) -> (5:w215:string, 7:w205:errorcluster)  [unwired: 2 in, 1 out]
                              n94 = Scan From String(format string="%.;%d", input string=w215) -> (output 1=w207:i32)  [unwired: 3 in, 3 out]
                              n95 = Equal?(x=w207, y=2) -> (x = y?=w216:bool)
                              n96 = Equal?(x=w207, y=6) -> (x = y?=w217:bool)
                              n97 = Or(x=w216, y=w217) -> (x .or. y?=w208:bool)
                            }
                          }
                          "CaptureStat" <- w197
                        }
                      }
                      frame #2 {
                        n98 = Number To Decimal String(number=w226) -> (decimal integer string=w243:string)  [unwired: 1 in]
                        n99 = Concatenate Strings("CAPTUREGET? " ("data"), "0" ("string"), "," ("string"), w243, ";" ("string")) -> (w245:string)
                        n100 = GPIB Write(0:w222, 1:w245, 3:w220) -> (6:w244:errorcluster)  [unwired: 2 in, 1 out]
                        n101 = GPIB Read(0:w222, 1:u32 2 ("byte count"), 3:w244) -> (5:w223:string, 7:w225:errorcluster)  [unwired: 2 in, 1 out]
                        "#n" <- w223
                        n102 = Scan From String(format string="#%d", input string=w223, error in=w225) -> (error out=w224:errorcluster, output 1=w241:i32)  [unwired: 1 in, 3 out]
                        "n" <- w241
                        n103 = GPIB Read(0:w222, 1:w241, 3:w224) -> (5:w235:string)  [unwired: 2 in, 2 out]
                        "cccc" <- w235
                        n104 = Scan From String(format string="%d", input string=w235) -> (output 1=w228:i32)  [unwired: 2 in, 4 out]
                        "number of bytes" <- w228
                        n105 = Increment(x=w228) -> (x+1=w229:i32)
                        n106 = GPIB Read(0:w222, 1:w229) -> (5:w221:string, 7:→"Error SR860":errorcluster)  [unwired: 3 in, 1 out]
                        "Buffer ASCII" <- w221
                        n107 = Unflatten From String(type=sgl[] [], binary string=w221, data includes array or string size? (T)=FALSE, byte order (0:big-endian, network order)=T6."little-endian") -> (value=w232:sgl[])  [unwired: 1 in, 2 out]
                        "Buffer" <- w232
                        n108 = Decimate 1D Array(w232) -> (w231:sgl[], w230:sgl[])
                        "R Buffer" <- w231
                        "Theta Buffer" <- w230
                        n109 = Array Size(array=w232) -> (size(s)=→"size(s)":i32)
                        n110 = call <vilib>:"Std Deviation and Variance.vi"("X"=w231) -> ("mean"=w219:dbl, "standard deviation"=w218:dbl)  [unwired: 1 in, 1 out]
                        n111 = local write "V Mean Now"(w219) -> ()
                        n112 = local write "V STD Now"(w218) -> ()
                        n113 = call <vilib>:"Std Deviation and Variance.vi"("X"=w230) -> ()  [unwired: 1 in, 3 out]
                      }
                    }
                  }
                  frame #1 {
                    # "Check if measured V is exceeding\nSCL or IRNG.\n\nIf yes, increment SCL by 10x\nIncrement RNG by 10x\n\nThen, measure voltage again"
                    n114 = local read "V Mean Now"() -> (w253:dbl)
                    n115 = local read "SCAL Now"() -> (w254:dbl)
                    n116 = local read "IRNG Now"() -> (w252:dbl)
                    n117 = Greater?(x=w253, y=w252) -> (0:w249:bool)
                    n118 = Greater Or Equal?(x=w253, y=w254) -> (x >= y?=w250:bool)
                    n119 = Or(x=w250, y=w249) -> (x .or. y?=w251:bool)
                    n120 = case shown="True" w251 {
                      tunnel: w256 -> [_ w260]
                      tunnel: w255 -> [_ w259]
                      tunnel: w250 -> [_ w258]
                      tunnel: w249 -> [_ w257]
                      frame False {
                      }
                      frame True {
                        n121 = stacked-sequence {
                          seq-local: [_ _ w303 _] -> [_ _ _ w340]
                          seq-local: [_ w299 _ _] -> [_ _ w302 _]
                          tunnel: w260 -> [w263 w301 w304 w341]
                          tunnel: w259 -> [_ _ _ w344]
                          tunnel: w258 -> [w264 _ _ _]
                          tunnel: w257 -> [w261 _ _ _]
                          frame #0 {
                            # "Change the IRNG and SCAL here"
                            n122 = flat-sequence {
                              tunnel: w264 -> [w267]
                              tunnel: w263 -> [w266]
                              tunnel: [w265] -> w262
                              tunnel: w262 -> [w284]
                              tunnel: w261 -> [w283]
                              frame #0 {
                                n123 = case shown="True" w267 {
                                tunnel: w266 -> [w268 w272]
                                tunnel: [w268 w272] -> w265
                                frame False {
                                }
                                frame True {
                                # "SCAL exceeded"
                                n124 = local read "Sensitivity"() -> (w281:T2)
                                n125 = Wait (ms)(milliseconds to wait=u32 1000) -> ()  [unwired: 1 out]
                                n126 = Subtract(x=w281, y=i16 3) -> (x-y=w279:u16)
                                n127 = Greater Than 0?(x=w279) -> (x > 0?=w280:bool)
                                n128 = Select(t=w279, s=w280, f=u16 0) -> (s? t:f=w271:u16)
                                n129 = local read "SCAL LUT"() -> (w270:dbl[])
                                n130 = local write "Sensitivity"(w271) -> ()
                                n131 = Number To Decimal String(number=w271) -> (decimal integer string=w276:string)  [unwired: 1 in]
                                n132 = Index Array(array=w270, index=w271) -> (element=w269:dbl)
                                n133 = local write "SCAL Now"(w269) -> ()
                                n134 = Concatenate Strings("SCAL " ("data"), w276, ";" ("string")) -> (w275:string)
                                n135 = GPIB Write(0:w272, 1:w275) -> ()  [unwired: 3 in, 2 out]
                                }
                                }
                              }
                              frame #1 {
                                n136 = case shown="True" w283 {
                                tunnel: w284 -> [_ w288]
                                frame False {
                                }
                                frame True {
                                # "IRNG exceeded"
                                n137 = local read "Input Range"() -> (w289:T1)
                                n138 = Wait (ms)(milliseconds to wait=u32 1000) -> ()  [unwired: 1 out]
                                n139 = Subtract(x=w289, y=i16 1) -> (x-y=w297:u16)
                                n140 = Greater Than 0?(x=w297) -> (x > 0?=w298:bool)
                                n141 = local read "IRNG LUT"() -> (w287:dbl[])
                                n142 = Select(t=w297, s=w298, f=u16 0) -> (s? t:f=w285:u16)
                                n143 = local write "Input Range"(w285) -> ()
                                n144 = Number To Decimal String(number=w285) -> (decimal integer string=w294:string)  [unwired: 1 in]
                                n145 = Index Array(array=w287, index=w285) -> (element=w286:dbl)
                                n146 = local write "IRNG Now"(w286) -> ()
                                n147 = Concatenate Strings("IRNG " ("data"), w294, ";" ("string")) -> (w293:string)
                                n148 = GPIB Write(0:w288, 1:w293) -> ()  [unwired: 3 in, 2 out]
                                }
                                }
                              }
                            }
                          }
                          frame #1 {
                            # "Start Buffer Acquistion"
                            n149 = GPIB Write(0:w301, 1:"CAPTURESTART ONE, IMM;" ("data")) -> (6:w299:errorcluster)  [unwired: 3 in, 1 out]
                          }
                          frame #2 {
                            # "Query the data capture state."
                            n150 = while {
                              tunnel: w304 -> [w309]
                              shift-right: [w306] -> w303
                              shift-left: w302 -> [w307]
                              stop <- w308 stop-if-true
                              # "Break loop when capture state is 2 or 6"
                              n151 = flat-sequence {
                                tunnel: w309 -> [w312]
                                tunnel: [w313] -> w310
                                tunnel: w307 -> [w311]
                                tunnel: w310 -> [w320]
                                tunnel: w309 -> [w322]
                                tunnel: [w318] -> w308
                                tunnel: [w317] -> w305
                                tunnel: [w315] -> w306
                                frame #0 {
                                n152 = GPIB Write(0:w312, 1:"CAPTURESTAT?;", 3:w311) -> (6:w313:errorcluster)  [unwired: 2 in, 1 out]
                                }
                                frame #1 {
                                n153 = Wait (ms)(milliseconds to wait=u32 50) -> ()  [unwired: 1 out]
                                n154 = GPIB Read(0:w322, 1:u32 4 ("byte count"), 3:w320) -> (5:w325:string, 7:w315:errorcluster)  [unwired: 2 in, 1 out]
                                n155 = Scan From String(format string="%.;%d", input string=w325) -> (output 1=w317:i32)  [unwired: 3 in, 3 out]
                                n156 = Equal?(x=w317, y=2) -> (x = y?=w326:bool)
                                n157 = Equal?(x=w317, y=6) -> (x = y?=w327:bool)
                                n158 = Or(x=w326, y=w327) -> (x .or. y?=w318:bool)
                                }
                              }
                              n159 = local write "CaptureStat"(w305) -> ()
                            }
                          }
                          frame #3 {
                            n160 = Number To Decimal String(number=w344) -> (decimal integer string=w353:string)  [unwired: 1 in]
                            n161 = Concatenate Strings("CAPTUREGET? " ("data"), "0" ("string"), "," ("string"), w353, ";" ("string")) -> (w355:string)
                            n162 = GPIB Write(0:w341, 1:w355, 3:w340) -> (6:w354:errorcluster)  [unwired: 2 in, 1 out]
                            n163 = GPIB Read(0:w341, 1:u32 2 ("byte count"), 3:w354) -> (5:w330:string, 7:w343:errorcluster)  [unwired: 2 in, 1 out]
                            n164 = Scan From String(format string="#%d", input string=w330, error in=w343) -> (error out=w342:errorcluster, output 1=w333:i32)  [unwired: 1 in, 3 out]
                            n165 = local write "#n"(w330) -> ()
                            n166 = local write "n"(w333) -> ()
                            n167 = GPIB Read(0:w341, 1:w333, 3:w342) -> (5:w329:string)  [unwired: 2 in, 2 out]
                            n168 = Scan From String(format string="%d", input string=w329) -> (output 1=w332:i32)  [unwired: 2 in, 4 out]
                            n169 = local write "cccc"(w329) -> ()
                            n170 = local write "number of bytes"(w332) -> ()
                            n171 = Increment(x=w332) -> (x+1=w346:i32)
                            n172 = GPIB Read(0:w341, 1:w346) -> (5:w337:string, 7:w328:errorcluster)  [unwired: 3 in, 1 out]
                            n173 = local write "Buffer ASCII"(w337) -> ()
                            n174 = local write "Error SR860"(w328) -> ()
                            n175 = Unflatten From String(type=sgl[] [], binary string=w337, data includes array or string size? (T)=FALSE, byte order (0:big-endian, network order)=T6."little-endian") -> (value=w336:sgl[])  [unwired: 1 in, 2 out]
                            n176 = local write "Buffer"(w336) -> ()
                            n177 = Decimate 1D Array(w336) -> (w334:sgl[], w335:sgl[])
                            n178 = Array Size(array=w336) -> (size(s)=w331:i32)
                            n179 = local write "R Buffer"(w334) -> ()
                            n180 = local write "size(s)"(w331) -> ()
                            n181 = local write "Theta Buffer"(w335) -> ()
                            n182 = call <vilib>:"Std Deviation and Variance.vi"("X"=w334) -> ("mean"=w339:dbl, "standard deviation"=w338:dbl)  [unwired: 1 in, 1 out]
                            n183 = local write "V Mean Now"(w339) -> ()
                            n184 = local write "V STD Now"(w338) -> ()
                            n185 = call <vilib>:"Std Deviation and Variance.vi"("X"=w335) -> ()  [unwired: 1 in, 3 out]
                          }
                        }
                      }
                    }
                  }
                }
              }
              frame #3 {
                # "Resistance"
                # "Voltage"
                # "Current"
                # "Write data to output array"
                n186 = local read "V Mean Now"() -> (w369:dbl)
                n187 = local read "Current Now"() -> (w376:string)
                n188 = local read "V STD Now"() -> (w367:dbl)
                n189 = Fract/Exp String To Number(string=w376) -> (number=w366:dbl)  [unwired: 3 in, 1 out]
                n190 = Divide(x=w369, y=w366) -> (x/y=w368:dbl)
                n191 = Divide(x=w367, y=w366) -> (x/y=w365:dbl)
                n192 = local read "Data array"() -> (w374:dbl[][])
                n193 = Build Array(w366, w369, w367, w368, w365) -> (w375:dbl[])
                n194 = Insert Into Array(array=w374, new element=w375) -> (w373:dbl[][])  [unwired: 2 in]
                n195 = local write "Data array"(w373) -> ()
                n196 = Index Array(array=w373, index (col) #1=0 ("index (row)"), index (col) #2=1 ("index (row)"), index (col) #3=3 ("index (col)")) -> (element #1=w363:dbl[], element #2=w372:dbl[], element #3=w362:dbl[])  [unwired: 3 in]
                n197 = Wait (ms)(milliseconds to wait=u32 100) -> ()  [unwired: 1 out]
                n198 = Bundle("Data array"=w363, "Data array"=w372) -> (w364:cluster{"Data array":dbl[], "Data array":dbl[]})  [unwired: 1 in]
                n199 = Bundle("Data array"=w363, "Data array"=w362) -> (w360:cluster{"Data array":dbl[], "Data array":dbl[]})  [unwired: 1 in]
                n200 = Build Array(w364, w360) -> (w359:T7)
                n201 = local write "I-V Plot"(w359) -> ()
              }
            }
          }
        }
      }
    }
    frame #4 {
      n202 = flat-sequence {
        tunnel: w378 -> [w381]
        frame #0 {
          n203 = Wait (ms)(milliseconds to wait=u32 1000) -> ()  [unwired: 1 out]
          n204 = GPIB Write(0:w381, 1:"SOURce:WAVE:ABORt" ("data")) -> ()  [unwired: 3 in, 2 out]
        }
        frame #1 {
          n205 = invoke class="VI" method="FP.Close"() -> ()  [unwired: 3 in, 3 out]
        }
      }
    }
  }
  n206 = case shown="\"Linear\", Default" "IV Sampling" {
    tunnel: "Ipts" -> [_ w415]
    tunnel: "Imax" -> [w389 w419]
    tunnel: "dI or Imin" -> [w382 w413]
    tunnel: "IV Type" -> [w393 _]
    frame "Linear", Default {
      n207 = Subtract(x=w389, y=w382) -> (x-y=w391:dbl)
      n208 = Multiply(x=w389, y=-1.0) -> (x*y=w388:dbl)
      n209 = call-poly <vilib>:"Ramp Pattern.vi"("start"=w382, "end"=w389, "delta"=w382) -> ("Ramp Pattern"=w392:dbl[])  [unwired: 6 in, 2 out]
      n210 = Add(x=w388, y=w382) -> (x+y=w387:dbl)
      n211 = Multiply(x=w382, y=-1.0) -> (x*y=w385:dbl)
      n212 = case shown="\"0 : Imax : 0\"" w393 {
        tunnel: w392 -> [w394 w399 w411]
        tunnel: [w394 w397 w409] -> w383
        tunnel: w391 -> [_ w400 w412]
        tunnel: w382 -> [_ w395 w406]
        tunnel: w388 -> [_ _ w404]
        tunnel: w387 -> [_ _ w408]
        tunnel: w385 -> [_ w396 w405]
        frame "0 : Imax", Default {
          # "For Linear sampling, possible to choose sweep type\n- Forward, 0:Imax\n-Half cycle, 0:Imax:0\n- Full cycles, 0:Imax:-Imax:0"
          # "Pass on the 0:Imax samples are they are"
        }
        frame "0 : Imax : 0" {
          n213 = call-poly <vilib>:"Ramp Pattern.vi"("start"=w400, "end"=w395, "delta"=w396) -> ("Ramp Pattern"=w398:dbl[])  [unwired: 6 in, 2 out]
          n214 = Insert Into Array(array=w399, new element=w398) -> (w397:dbl[])  [unwired: 1 in]
        }
        frame "0 : Imax : -Imax : 0" {
          n215 = call-poly <vilib>:"Ramp Pattern.vi"("start"=w412, "end"=w406, "delta"=w405) -> ("Ramp Pattern"=w410:dbl[])  [unwired: 6 in, 2 out]
          n216 = Insert Into Array(array=w411, new element=w410) -> (w403:dbl[])  [unwired: 1 in]
          n217 = call-poly <vilib>:"Ramp Pattern.vi"("start"=w405, "end"=w404, "delta"=w405) -> ("Ramp Pattern"=w401:dbl[])  [unwired: 6 in, 2 out]
          n218 = Insert Into Array(array=w403, new element=w401) -> (w402:dbl[])  [unwired: 1 in]
          n219 = call-poly <vilib>:"Ramp Pattern.vi"("start"=w408, "end"=w405, "delta"=w406) -> ("Ramp Pattern"=w407:dbl[])  [unwired: 6 in, 2 out]
          n220 = Insert Into Array(array=w402, new element=w407) -> (w409:dbl[])  [unwired: 1 in]
        }
      }
      n221 = local write "Current Samples"(w383) -> ()
      n222 = Array Size(array=w383) -> (size(s)=w384:i32)
      n223 = local write "Ipts"(w384) -> ()
    }
    frame "Logartihmic" {
      n224 = Divide(x=w419, y=w413) -> (x/y=w418:dbl)
      n225 = Decrement(x=w415) -> (x-1=w416:i16)
      n226 = Logarithm Base 10(1:w418) -> (0:w417:dbl)
      n227 = Divide(x=w417, y=w416) -> (x/y=w414:dbl)
      n228 = for {
        N: w415 -> [_]
        tunnel: w414 -> [w425]
        tunnel: w413 -> [w421]
        i -> [w424]
        n229 = local read "Current Samples"() -> (w426:dbl[])
        n230 = Multiply(x=w425, y=w424) -> (x*y=w423:dbl)
        n231 = Power Of 10(x=w423) -> (10^x=w422:dbl)
        n232 = Multiply(x=w421, y=w422) -> (x*y=w420:dbl)
        n233 = Insert Into Array(array=w426, new element=w420) -> (w427:dbl[])  [unwired: 1 in]
        n234 = local write "Current Samples"(w427) -> ()
      }
    }
  }
  "Current Samples" <- dbl[] [] ("array")
  "IRNG LUT" <- dbl[] [1.0, 0.3, 0.1, 0.03, 0.01] ("array")
  "SCAL LUT" <- dbl[] [1.0, 0.5, 0.2, 0.1, 0.05, 0.02, 0.01, 0.005, 0.002, 0.001, 0.0005, 0.0002, 0.0001, 5e-05, 2e-05, 1e-05, 5e-06, 2e-06, 1e-06, 5e-07, 2e-07, 1e-07, 5e-08, 2e-08, 1e-08, 5e-09, 2e-09, 1e-09] ("array")
  "OFLT LUT" <- dbl[] [1e-06, 3e-06, 1e-05, 3e-05, 0.0001, 0.0003, 0.001, 0.003, 0.01, 0.03, 0.1, 0.3, 1.0, 3.0, 10.0, 30.0, 100.0, 300.0, 1000.0, 3000.0, 10000.0, 30000.0] ("array")
  "Data array" <- dbl[][] [] ("Data array")
